vi "Pass if Result.vi"(8 "error in (no error)":errorcluster, 9 "timeout in ms (0)":i32, 11 "Test Runner Test in":refnum<class "Test Runner Test.lvclass">) -> (0 "error out":errorcluster, 3 "Test Runner Test out":refnum<class "Test Runner Test.lvclass">)   [LabVIEW 2020, in "Test Runner Test.lvclass"]
uses:
  Test Runner Test.lvclass
  Test Runner Test.lvclass/Test Runner Test.ctl
  <vilib>/Astemes/LUnit/Test Case.lvclass
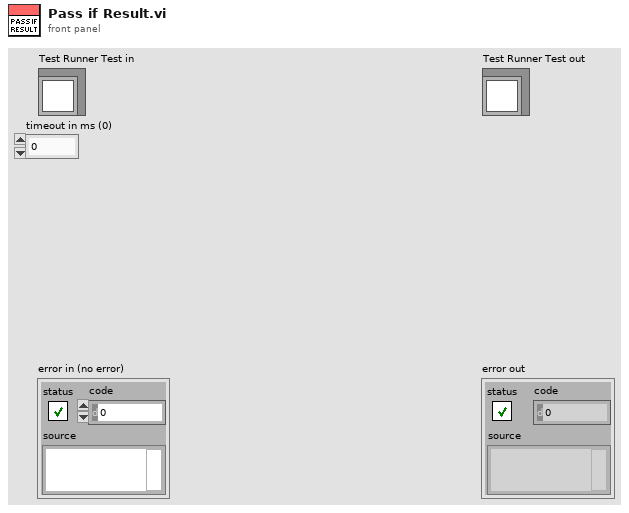
[diagram p1: front panel]
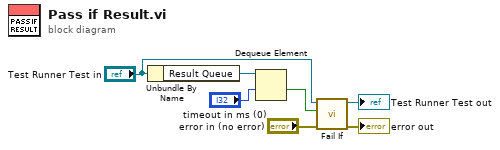
[diagram p0: block diagram]
diagram:
  n1 = Unbundle By Name("Test Runner Test in") -> ("Result Queue"=w6:refnum<queue>)
  n2 = Dequeue Element(queue=w6, timeout in ms (-1)="timeout in ms (0)") -> (timed out?=w3:bool)  [unwired: 1 in, 3 out]
  n3 = call <vilib>:"Fail If.vi"("error in (no error)"="error in (no error)", "Fail?"=w3, "LUnit Test Case In"="Test Runner Test in") -> ("error out"=→"error out":errorcluster, "LUnit Test Case Out"=→"Test Runner Test out":refnum<class "Test Runner Test.lvclass">)  [unwired: 7 in]
